vi "Engine.vi"(8 "error in (no error)":errorcluster, 11 "Message Queue":refnum<queue>) -> (0 "error out":errorcluster)   [LabVIEW 2018, in "Module.lvclass"]
uses:
  Module.lvclass
  support/Message Queue/Message Cluster.ctl
  support/Message Queue/Enqueue Message (Single).vi
  support/Message Queue/Message Queue.lvlib
panel:
  out "Instance Name":string
  in  "Exit":bool
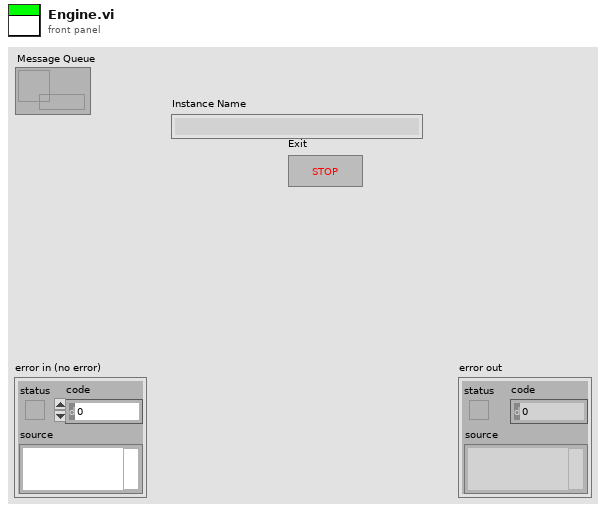
[diagram p1: front panel]
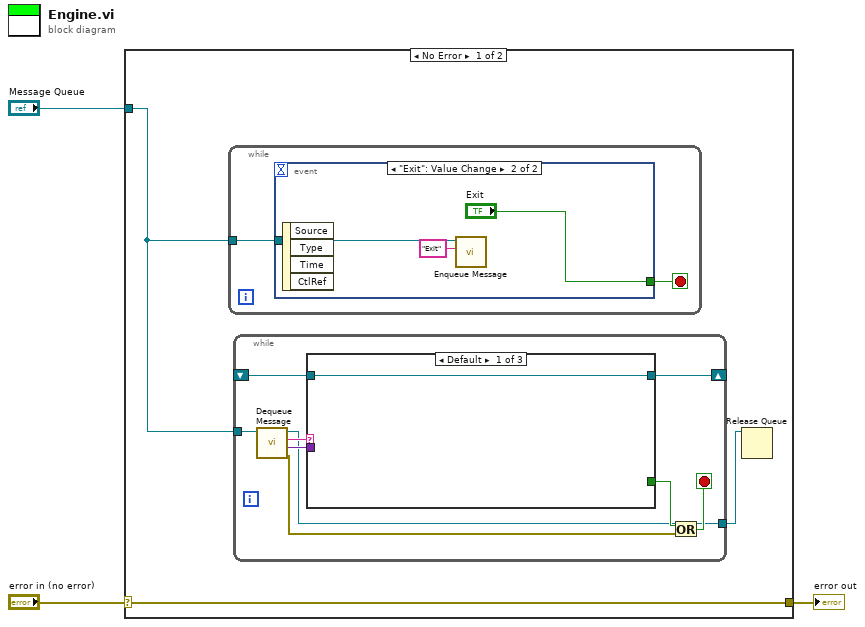
[diagram p0: block diagram]
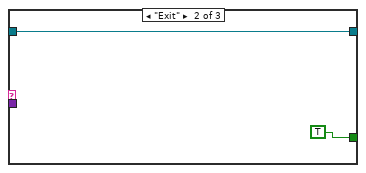
[diagram p2: hidden frame]
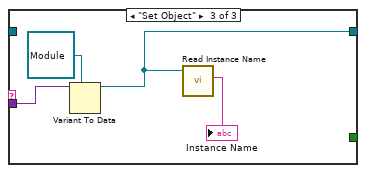
[diagram p3: hidden frame]
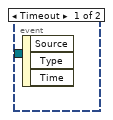
[diagram p4: hidden frame]
diagram:
  n1 = case shown="No Error" "error in (no error)" {
    selector: "error in (no error)" -> [w6 w28]
    tunnel: [w6 w28] -> w2
    tunnel: "Message Queue" -> [w5 _]
    frame No Error {
      n2 = while {
        tunnel: w5 -> [w23]
        stop <- w24 stop-if-true
        n3 = event shown="[1] \"Exit\": Value Change" {
          selector: _ -> [_ _]
          dyn-events: _ -> [_ _]
          timeout: _ -> [_ _]
          tunnel: [_ "Exit"] -> w24
          tunnel: w23 -> [_ w26]
          event Timeout {
            n4 = event-data() -> ()  [unwired: 1 in, 3 out]
          }
          event "Exit": Value Change {
            n5 = event-data() -> ()  [unwired: 1 in, 4 out]
            n6 = call-poly "Enqueue Message.vi"("Message"="Exit", "Message Queue"=w26) -> ()  [unwired: 8 in, 2 out]
          }
        }
      }
      n7 = while {
        shift-right: [w12] -> _
        shift-left: _ -> [w11]
        tunnel: w5 -> [w15]
        tunnel: [w7] -> w4
        stop <- w8 stop-if-true
        n8 = call "Dequeue Message.vi"("Message Queue"=w15) -> ("error out"=w10:errorcluster, "Message Data"=w13:variant, "Message"=w14:string, "dup Message Queue"=w7:refnum<queue>)  [unwired: 7 in]
        n9 = case shown="Default" w14 {
          tunnel: w13 -> [_ _ w21]
          tunnel: [w16 w18 w19] -> w12
          tunnel: w11 -> [w16 w18 _]
          tunnel: [_ TRUE _] -> w9
          frame Default {
          }
          frame "Exit" {
          }
          frame "Set Object" {
            n10 = Variant To Data(type=refnum<class "Module.lvclass"> refnum ("Module out"), Variant=w21) -> (data=w19:refnum<class "Module.lvclass">)  [unwired: 1 in, 1 out]
            n11 = call-dynamic "Read Instance Name.vi"("Module in"=w19) -> ("Instance Name"=→"Instance Name":string)  [unwired: 8 in, 2 out]
          }
        }
        n12 = Or(x=w9, y=w10) -> (x .or. y?=w8:bool)
      }
      n13 = Release Queue(queue=w4) -> ()  [unwired: 2 in, 3 out]
    }
    frame Error {
    }
  }
  "error out" <- w2
